vi "Set ILC.vi"(10 "HPILC":refnum<class "HPILC.lvclass">, 11 "Model in":refnum<class "Model.lvclass">) -> (3 "Model out":refnum<class "Model.lvclass">)   [LabVIEW 2016, in "Model.lvclass"]
uses:
  Model.lvclass
  common_rt_hpilc/HPILC/HPILC.lvclass
  C:/CODE/ts_hpmt/common_rt_ilc/ILC/ILC.lvclass
  Model.lvclass/Model.ctl
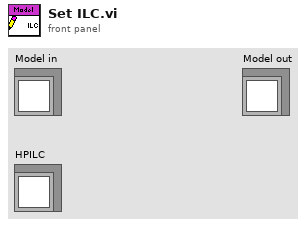
[diagram p1: front panel]
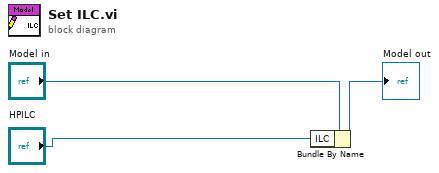
[diagram p0: block diagram]
diagram:
  n1 = Bundle By Name(cluster="Model in", "ILC"="HPILC") -> (→"Model out":refnum<class "Model.lvclass">)
